vi "ImageExtraction.vi"() -> ()   [LabVIEW 2015]
uses:
  <vilib>/Analysis/NI_AALBase.lvlib
panel:
  out "Modified Angle":dbl[](array[numeric])
  in  "Tab Control":enum32{"Analysis", "Extracted Data"}(tab)
  out "Progress":bool
  out "Improved Threshold":T1(plugin-control)
  in  "Extract Data":bool
  in  "Method":i32(ring) items=["Niblack", "Background Correction", "Constant Threshold", "Auto Threshold"]
  in  "Parameters":T2={"Look for"=1, "Window Size"={"X axis"=72, "Y axis"=72}, "Niblack\nDeviation\nFactor"=1.0, "Threshold"={169, 221}, "No of erosion"=2} {"Threshold" scale=0.0..255.0; "Niblack\nDeviation\nFactor" min=0.0 max=1.0 step=0.01 format="%.2f"; "Look for" items=["Bright Objects", "Dark Objects"]}
  out "Clamped Image":T1(plugin-control)
  out "Threshold Image":T1(plugin-control)
  in  "File Type":bool
  out "File Path":path
  out "Original":T1(plugin-control)
  in  "Frame":i32(slide) min=0 max=3507 step=1 scale=0.0..3507.0 scale format="%1.0f"
  in  "Stop Button":bool
  in  "Set starting Frame":bool
  out "Starting Frame":i32
  in  "Set final frame":bool
  out "Final Frame":i32
  out "Length Array":dbl[](array[numeric])
  out "Frame No":i32[](array[numeric])
  out "Unmodified Angle":dbl[](array[numeric])
  in  "Extract Length":bool
  out "Length Extraction":T3
  out "Length":cluster{i32[], dbl[]}(graph)
  out "Off Plane Angle":cluster{i32[], dbl[]}(graph)
  out "Mean":dbl format="%0.2f"
  out "Standard Deviation":dbl format="%0.2f"
  out "Variance":dbl format="%0.2f"
  out "In-plane Angle":cluster{i32[], dbl[]}(graph)
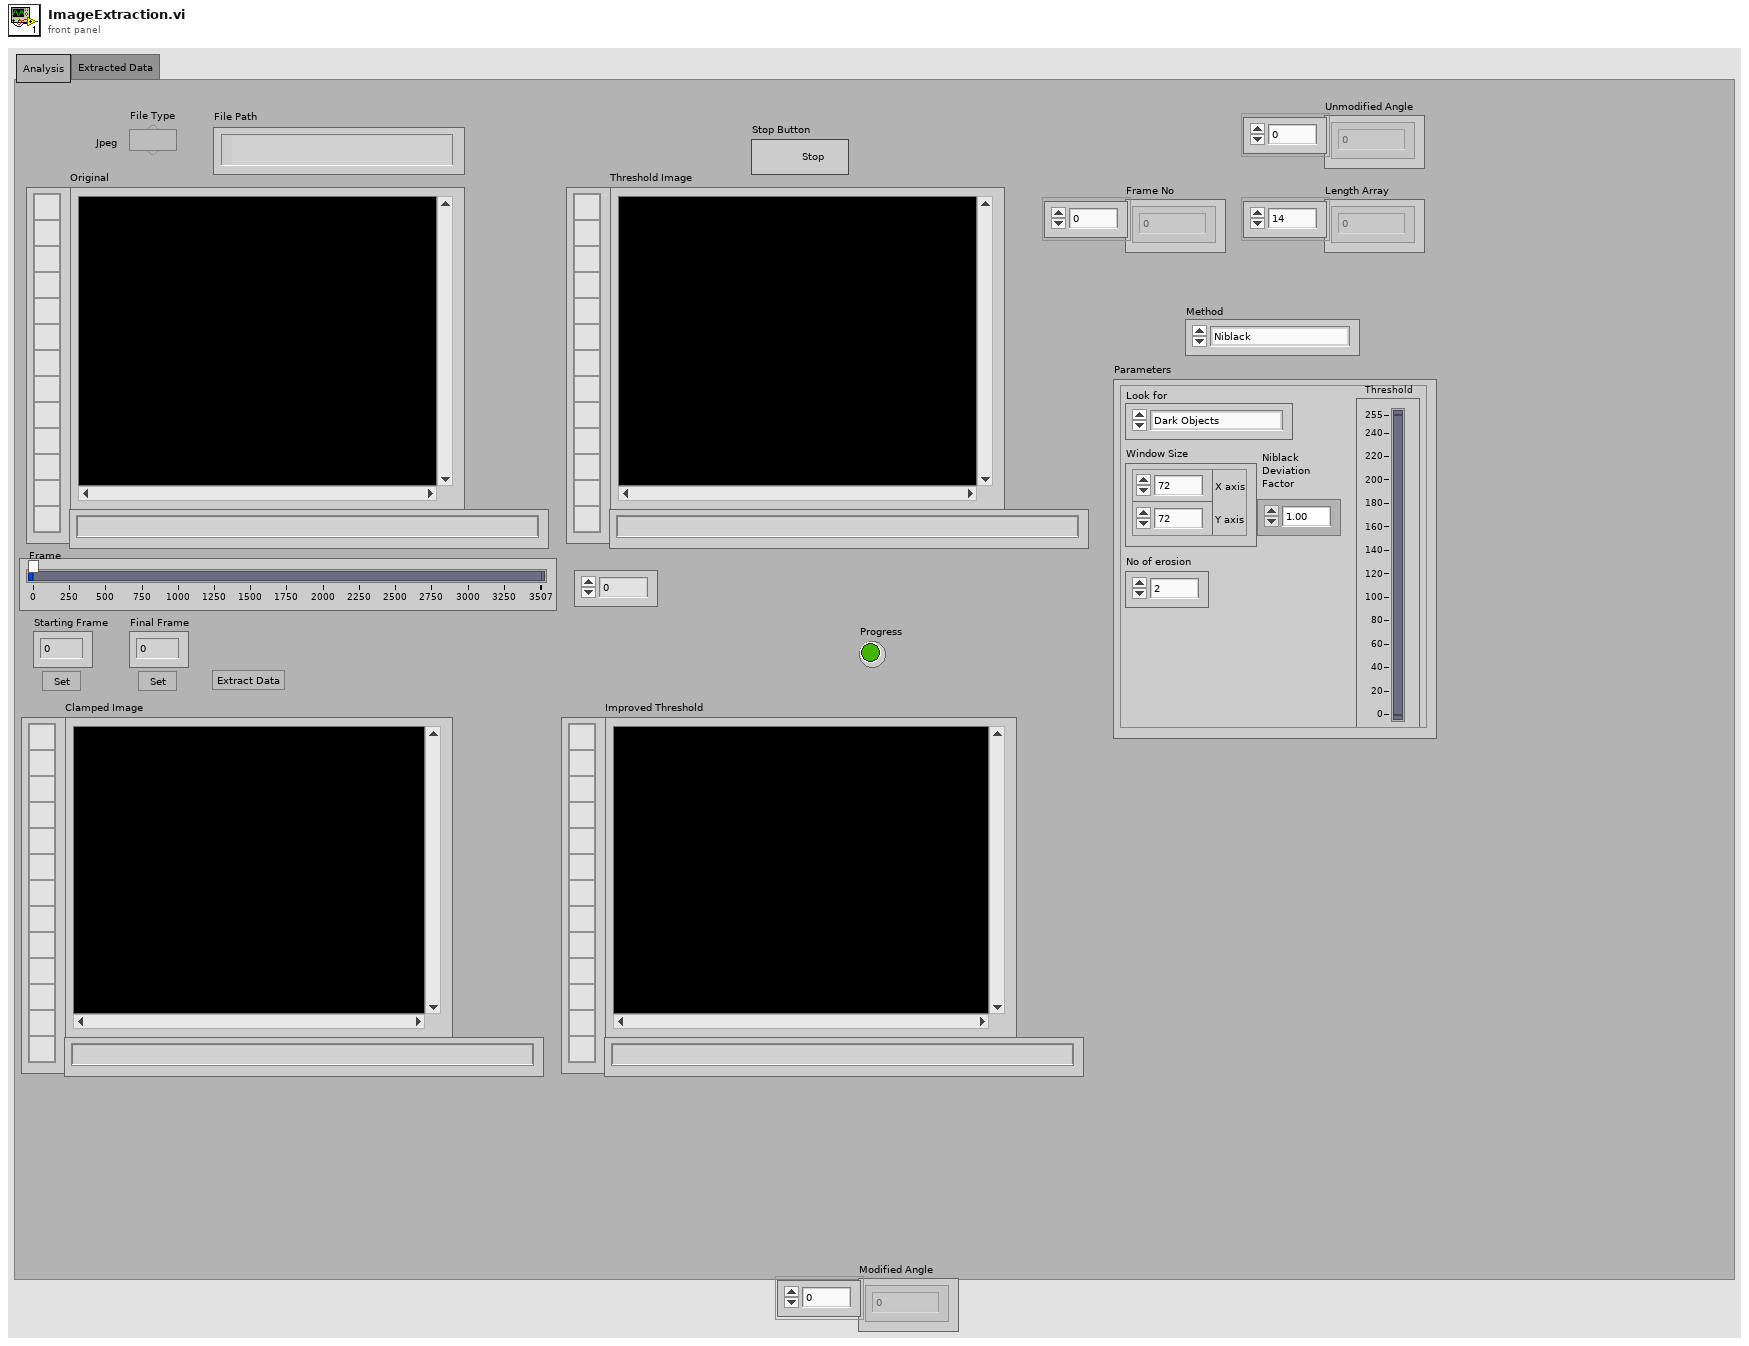
[diagram p1: front panel]
types:
  T1 = typedef "IMAQ Image.ctl" = refnum<image>
  T2 = cluster{"Look for":i32, "Window Size":cluster{"X axis":i32, "Y axis":i32}, "Niblack\nDeviation\nFactor":dbl, "Threshold":cluster{i32, i32}, "No of erosion":i32}
  T3 = cluster{"Initial":cluster{"Initial Frame":u32, "Initial Length":u32}, "Final":cluster{"Final Frame":u32, "Final Length":u32}}
  T4 = cluster{"Global Rectangle":i32[], "Contours":cluster{"Contour Type":u32, "ROI Type":u32, "Points":i32[]}[]}
  T5 = typedef "ROI Descriptor" = cluster{"Global Rectangle":i32[], "Contours":cluster{"ID":enum32{"External", "Internal"}, "Type":u32, "Coordinates":i32[]}[]}
  T6 = cluster{"Distance (Pixels)":dbl, "Distance (Real World)":dbl, "Angle (Absolute)":dbl, "Angle (Relative)":dbl}
  T7 = typedef "LVPointDoubleTypeDef.ctl" = cluster{"Cursor X":dbl, "Cursor Y":dbl}
  T8 = cluster{"Cursor.Cursor Position":T7, "Cursor.Cursor Position":T7}
  T9 = cluster{"Initial Frame":u32, "Initial Length":u32}
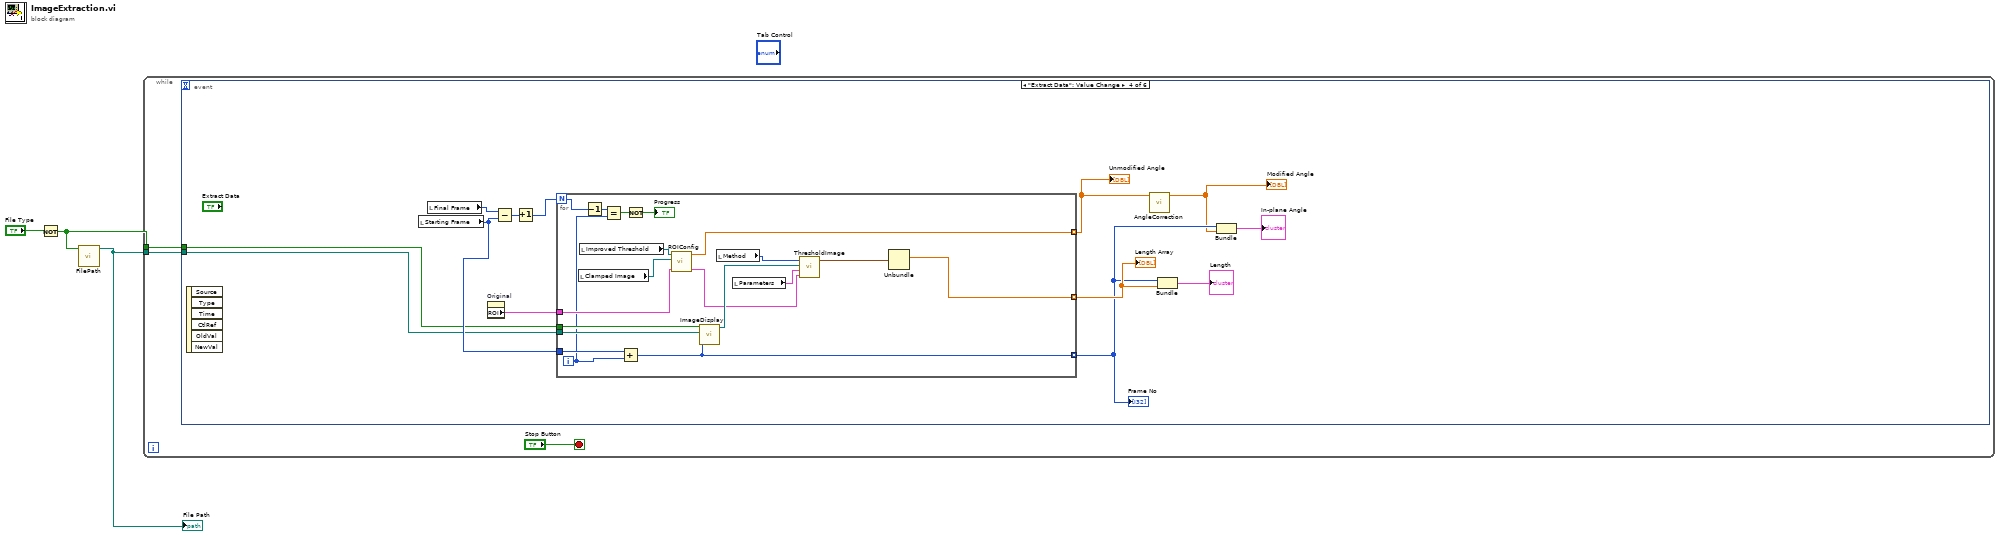
[diagram p0: block diagram]
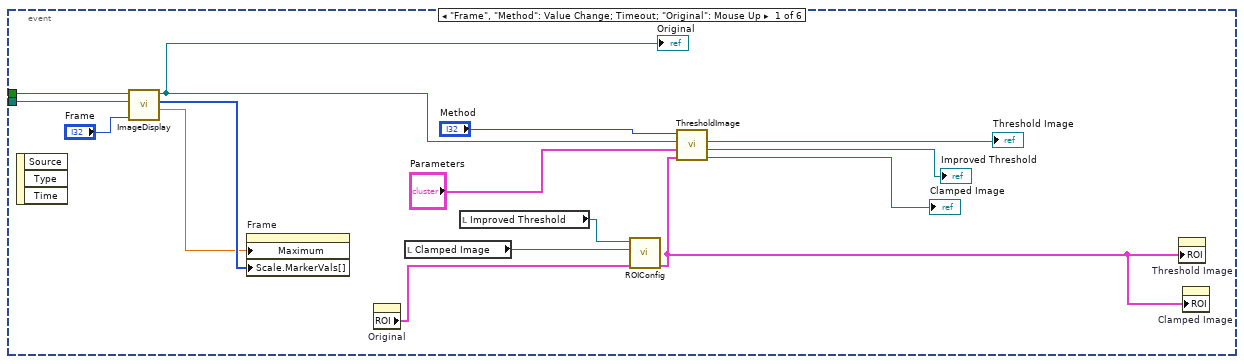
[diagram p2: hidden frame]
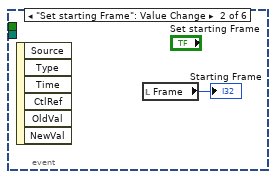
[diagram p3: hidden frame]
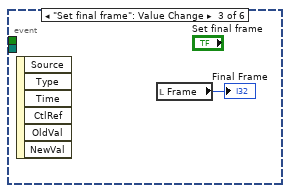
[diagram p4: hidden frame]
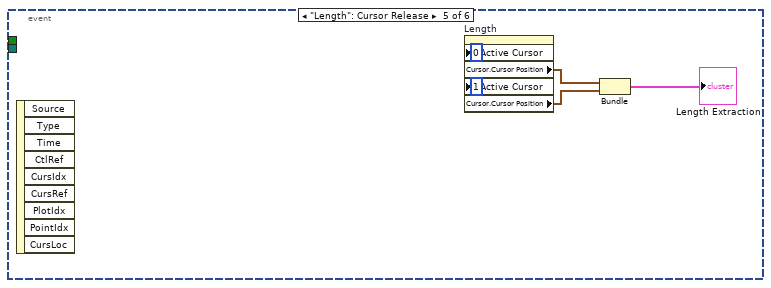
[diagram p5: hidden frame]
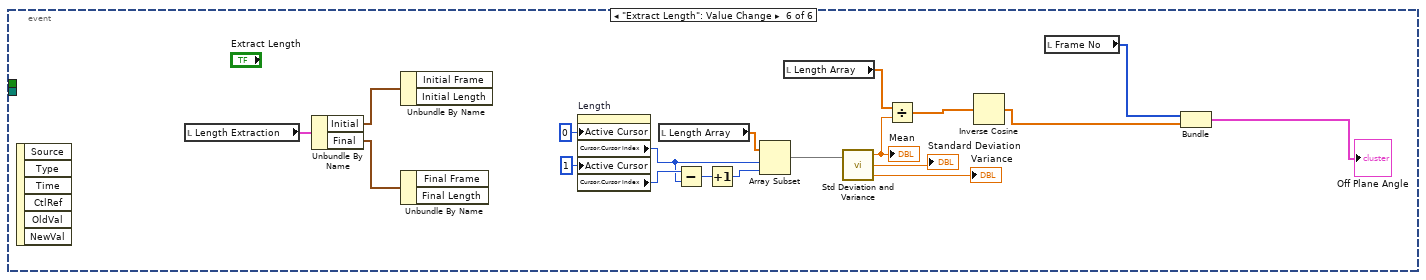
[diagram p6: hidden frame]
diagram:
  n1 = Not(x="File Type") -> (.not. x?=w1:bool)
  n2 = call "FilePath.vi"("Boolean"=w1) -> ("Path"=w2:path)  [unwired: 10 in]
  "File Path" <- w2
  n3 = while {
    tunnel: w2 -> [w4]
    tunnel: w1 -> [w5]
    stop <- "Stop Button" stop-if-true
    n4 = event shown="[3] \"Extract Data\": Value Change" {
      selector: _ -> [_ _ _ _ _ _]
      dyn-events: _ -> [_ _ _ _ _ _]
      timeout: _ -> [_ _ _ _ _ _]
      tunnel: w5 -> [w18 _ _ w30 _ _]
      tunnel: w4 -> [w17 _ _ w29 _ _]
      event "Parameters.Threshold", "Frame", "Method", "Parameters.Look for", "Parameters.Niblack\nDeviation\nFactor", "Parameters.No of erosion": Value Change; Timeout; "Original": Mouse Up {
        n5 = event-data() -> ()  [unwired: 1 in, 3 out]
        n6 = call "ImageDisplay.vi"("Frame"="Frame", "Path"=w17, "JPG or AVI"=w18) -> ("Number of frames"=w19:dbl, "Frames"=w20:u32[], "Image"=w13:T1)  [unwired: 5 in]
        "Original" <- w13
        n7 = property on="Frame" class="Slide (strict)"("Maximum"=w19, "Scale.MarkerVals[]"=w20) -> ()  [unwired: 2 in, 2 out]
        n8 = property on="Original" class="ImageControl"() -> ("ROI"=w10:T4)  [unwired: 2 in, 2 out]
        n9 = local read "Clamped Image"() -> (w8:T1)
        n10 = local read "Improved Threshold"() -> (w9:T1)
        n11 = call "ROIConfig.vi"("ROI In"=w10, "Clamped Image"=w8, "Improved threshold"=w9) -> ("ROI  Out"=w7:T5)  [unwired: 7 in, 1 out]
        n12 = call "ThresholdImage.vi"("Method"="Method", "Image Src"=w13, "Cluster"="Parameters", "ROI Descriptor"=w7) -> ("Threshold"=→"Threshold Image":T1, "Improved Threshold"=→"Improved Threshold":T1, "Clamped Image"=→"Clamped Image":T1)  [unwired: 3 in, 1 out]
        n13 = property on="Threshold Image" class="ImageControl"("ROI"=w7) -> ()  [unwired: 2 in, 2 out]
        n14 = property on="Clamped Image" class="ImageControl"("ROI"=w7) -> ()  [unwired: 2 in, 2 out]
      }
      event "Set starting Frame": Value Change {
        n15 = event-data() -> ()  [unwired: 1 in, 6 out]
        n16 = local read "Frame"() -> (→"Starting Frame":i32)
      }
      event "Set final frame": Value Change {
        n17 = event-data() -> ()  [unwired: 1 in, 6 out]
        n18 = local read "Frame"() -> (→"Final Frame":i32)
      }
      event "Extract Data": Value Change {
        n19 = event-data() -> ()  [unwired: 1 in, 6 out]
        n20 = local read "Starting Frame"() -> (w33:i32)
        n21 = local read "Final Frame"() -> (w36:i32)
        n22 = property on="Original" class="ImageControl"() -> ("ROI"=w34:T4)  [unwired: 2 in, 2 out]
        n23 = Subtract(x=w36, y=w33) -> (x-y=w35:i32)
        n24 = Increment(x=w35) -> (x+1=w28:i32)
        n25 = for {
          N: w28 -> [w40]
          tunnel: [w42] -> w31 mode=indexing
          tunnel: w34 -> [w45]
          tunnel: w33 -> [w55]
          tunnel: [w54] -> w27 mode=indexing
          tunnel: w30 -> [w53]
          tunnel: w29 -> [w52]
          tunnel: [w43] -> w24 mode=indexing
          i -> [w38]
          n26 = local read "Clamped Image"() -> (w47:T1)
          n27 = local read "Improved Threshold"() -> (w46:T1)
          n28 = Decrement(x=w40) -> (x-1=w39:i32)
          n29 = Equal?(x=w39, y=w38) -> (x = y?=w37:bool)
          n30 = Add(x=w55, y=w38) -> (x+y=w54:i32)
          n31 = Not(x=w37) -> (.not. x?=→"Progress":bool)
          n32 = call "ROIConfig.vi"("ROI In"=w45, "Clamped Image"=w47, "Improved threshold"=w46) -> ("ROI  Out"=w44:T5, "Orientation"=w43:dbl)  [unwired: 7 in]
          n33 = call "ImageDisplay.vi"("Frame"=w54, "Path"=w52, "JPG or AVI"=w53) -> ("Image"=w50:T1)  [unwired: 5 in, 2 out]
          n34 = local read "Method"() -> (w49:i32)
          n35 = local read "Parameters"() -> (w51:T2)
          n36 = call "ThresholdImage.vi"("Method"=w49, "Image Src"=w50, "Cluster"=w51, "ROI Descriptor"=w44) -> ("Clamp Results"=w48:T6)  [unwired: 3 in, 3 out]
          n37 = Unbundle(w48) -> ("Distance (Real World)"=w42:dbl)  [unwired: 3 out]
        }
        "Length Array" <- w31
        "Frame No" <- w27
        "Unmodified Angle" <- w24
        n38 = call "AngleCorrection.vi"("Oiiginal"=w24) -> ("Modified"=w25:dbl[])  [unwired: 10 in]
        "Modified Angle" <- w25
        n39 = Bundle(w27, w31) -> (→"Length":cluster{i32[], dbl[]})  [unwired: 1 in]
        n40 = Bundle(w27, "Modified"=w25) -> (→"In-plane Angle":cluster{i32[], "Modified":dbl[]})  [unwired: 1 in]
      }
      event "Length": Cursor Release {
        n41 = event-data() -> ()  [unwired: 1 in, 9 out]
        n42 = property on="Length" class="XYGraph (strict)"("Active Cursor"=u32 0, "Active Cursor"=u32 1) -> ("Cursor.Cursor Position"=w58:T7, "Cursor.Cursor Position"=w57:T7)  [unwired: 2 in, 2 out]
        n43 = Bundle("Cursor.Cursor Position"=w58, "Cursor.Cursor Position"=w57) -> (→"Length Extraction":T8)  [unwired: 1 in]
      }
      event "Extract Length": Value Change {
        n44 = event-data() -> ()  [unwired: 1 in, 6 out]
        n45 = local read "Length Extraction"() -> (w79:T3)
        n46 = Unbundle By Name(w79) -> ("Initial"=w78:T9, "Final"=w77:cluster{"Final Frame":u32, "Final Length":u32})
        n47 = Unbundle By Name(w78) -> ()  [unwired: 2 out]
        n48 = Unbundle By Name(w77) -> ()  [unwired: 2 out]
        n49 = property on="Length" class="XYGraph (strict)"("Active Cursor"=u32 0, "Active Cursor"=u32 1) -> ("Cursor.Cursor Index"=w69:i32, "Cursor.Cursor Index"=w70:i32)  [unwired: 2 in, 2 out]
        n50 = local read "Length Array"() -> (w72:dbl[])
        n51 = Subtract(x=w70, y=w69) -> (x-y=w74:i32)
        n52 = Increment(x=w74) -> (x+1=w73:i32)
        n53 = Array Subset(array=w72, index=w69, length=w73) -> (w71:dbl[])
        n54 = local read "Length Array"() -> (w65:dbl[])
        n55 = call <vilib>:"Std Deviation and Variance.vi"("X"=w71) -> ("mean"=w66:dbl, "standard deviation"=→"Standard Deviation":dbl, "variance"=→"Variance":dbl)  [unwired: 1 in]
        "Mean" <- w66
        n56 = Divide(x=w65, y=w66) -> (x/y=w64:dbl[])
        n57 = Inverse Cosine(1:w64) -> (0:w62:dbl[])
        n58 = local read "Frame No"() -> (w63:i32[])
        n59 = Bundle("Frame No"=w63, w62) -> (→"Off Plane Angle":cluster{"Frame No":i32[], dbl[]})  [unwired: 1 in]
      }
    }
  }
